vi "Test Assert Equal Value (Arrays).vi"(8 "error in (no error)":errorcluster) -> (0 "error out":errorcluster)   [LabVIEW 2009]
uses:
  classes/Assert/Assert.lvclass
  classes/Test/Test.lvclass
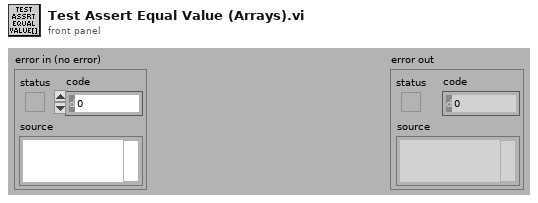
[diagram p1: front panel]
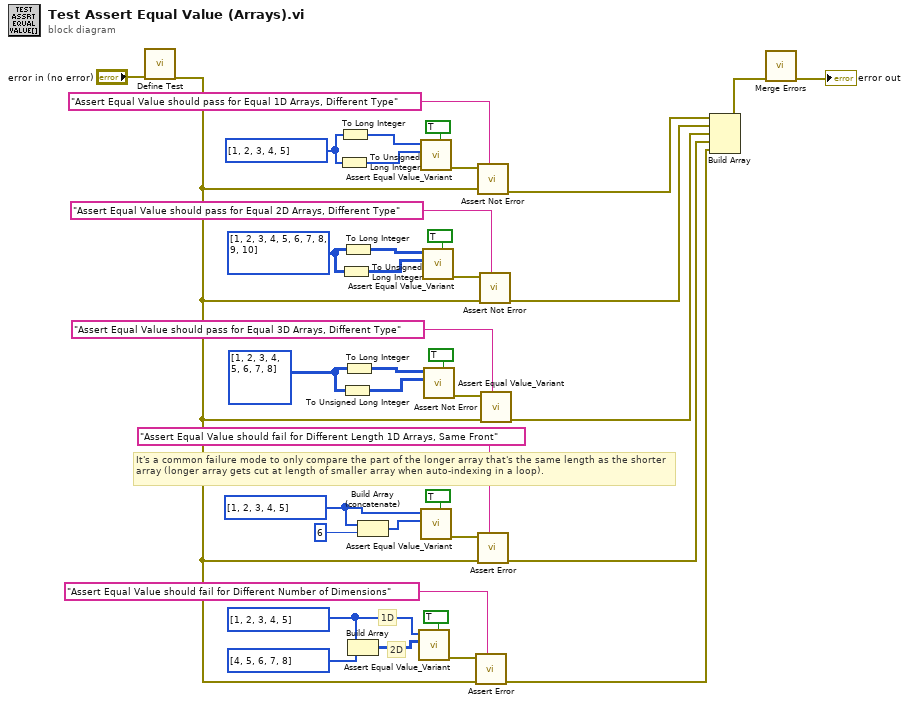
[diagram p0: block diagram]
diagram:
  w1 = u64[] [1, 2, 3, 4, 5]
  w14 = u64[] [1, 2, 3, 4, 5]
  w19 = i32[][][] [[[1, 2], [3, 4]], [[5, 6], [7, 8]]]
  w27 = u64[][] [[1, 2, 3, 4, 5], [6, 7, 8, 9, 10]]
  w32 = u64[] [1, 2, 3, 4, 5]
  # "2D"
  # "1D"
  # "It's a common failure mode to only compare the part of the longer array that's the same length as the shorter array (longer array gets cut at length of smaller array when auto-indexing in a loop)."
  n1 = call "Define Test.vi"("error in (no error)"="error in (no error)") -> ("error out"=w5:errorcluster)  [unwired: 10 in]
  n2 = To Unsigned Long Integer(number=w32) -> (unsigned 32bit integer=w30:u32[])
  n3 = To Long Integer(number=w32) -> (32bit integer=w31:i32[])
  n4 = To Unsigned Long Integer(number=w27) -> (unsigned 32bit integer=w29:u32[][])
  n5 = To Unsigned Long Integer(number=w19) -> (unsigned 32bit integer=w17:u32[][][])
  n6 = To Long Integer(number=w27) -> (32bit integer=w28:i32[][])
  n7 = To Long Integer(number=w19) -> (32bit integer=w18:i32[][][])
  n8 = Build Array(w1, u64[] [4, 5, 6, 7, 8]) -> (w2:u64[][])
  n9 = Build Array (concatenate)(w14, u64 6) -> (w12:u64[])
  n10 = call "Assert Equal Value_Variant.vi"("Assert Only? (F)"=TRUE, "Y"=w2, "X"=w1) -> ("error out"=w8:errorcluster)  [unwired: 8 in]
  n11 = call "Assert Equal Value_Variant.vi"("Assert Only? (F)"=TRUE, "Y"=w30, "X"=w31) -> ("error out"=w35:errorcluster)  [unwired: 8 in]
  n12 = call "Assert Equal Value_Variant.vi"("Assert Only? (F)"=TRUE, "Y"=w12, "X"=w14) -> ("error out"=w10:errorcluster)  [unwired: 8 in]
  n13 = call "Assert Equal Value_Variant.vi"("Assert Only? (F)"=TRUE, "Y"=w29, "X"=w28) -> ("error out"=w25:errorcluster)  [unwired: 8 in]
  n14 = call "Assert Equal Value_Variant.vi"("Assert Only? (F)"=TRUE, "Y"=w17, "X"=w18) -> ("error out"=w21:errorcluster)  [unwired: 8 in]
  n15 = call "Assert Error.vi"("Label"="Assert Equal Value should fail for Different Number of Dimensions", "error in (no error)"=w5, "Error?"=w8) -> ("error out"=w4:errorcluster)  [unwired: 8 in]
  n16 = call "Assert Not Error.vi"("Label"="Assert Equal Value should pass for Equal 1D Arrays, Different Type", "error in (no error)"=w5, "Not Error?"=w35) -> ("error out"=w33:errorcluster)  [unwired: 8 in]
  n17 = call "Assert Error.vi"("Label"="Assert Equal Value should fail for Different Length 1D Arrays, Same Front", "error in (no error)"=w5, "Error?"=w10) -> ("error out"=w9:errorcluster)  [unwired: 8 in]
  n18 = call "Assert Not Error.vi"("Label"="Assert Equal Value should pass for Equal 2D Arrays, Different Type", "error in (no error)"=w5, "Not Error?"=w25) -> ("error out"=w23:errorcluster)  [unwired: 8 in]
  n19 = call "Assert Not Error.vi"("Label"="Assert Equal Value should pass for Equal 3D Arrays, Different Type", "error in (no error)"=w5, "Not Error?"=w21) -> ("error out"=w16:errorcluster)  [unwired: 8 in]
  n20 = Build Array(w33, w23, w16, w9, w4) -> (w37:errorcluster[])
  n21 = call <vilib>:"Merge Errors.vi"("error array in"=w37) -> ("error out"=→"error out":errorcluster)  [unwired: 6 in]
